vi "Gill_get_rdg.vi"(4 "Channel Name":string, 7 "Address":T1={"Main"=67, "Ch."=2, "Sub"=982, "Port Name"="Printer-Modem Port"}) -> (0 "Output":dbl format="%.2f", 3 "Status note":string)   [LabVIEW 2010]
uses:
  ADAM Client/Sub VIs/ADAM Controls/Address.ctl
  ADAM Client/Sub VIs/ADAM Controls/Remember_value_mode.ctl
panel:
  out "Concatenated String":string
  out "4521 Address":string
  out "Gill type":i32
  out "ADDRESS LETTER":string
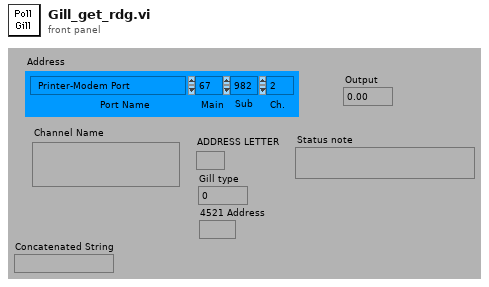
[diagram p1: front panel]
types:
  T1 = typedef "Address.ctl" = cluster{"Main":i32, "Ch.":i32, "Sub":i32, "Port Name":string}
  T2 = typedef "Remember_value_mode.ctl" = enum16{"Read only", "Read and Write"}
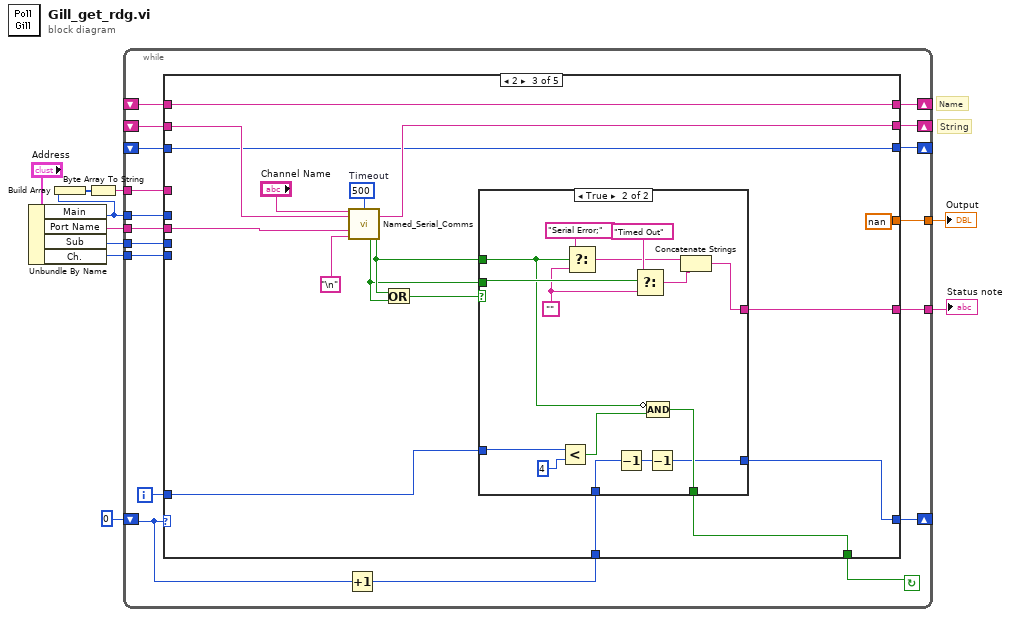
[diagram p0: block diagram]
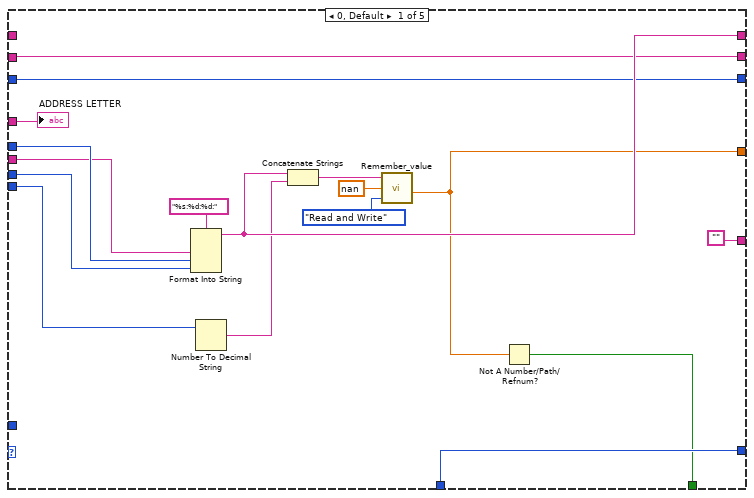
[diagram p2: hidden frame]
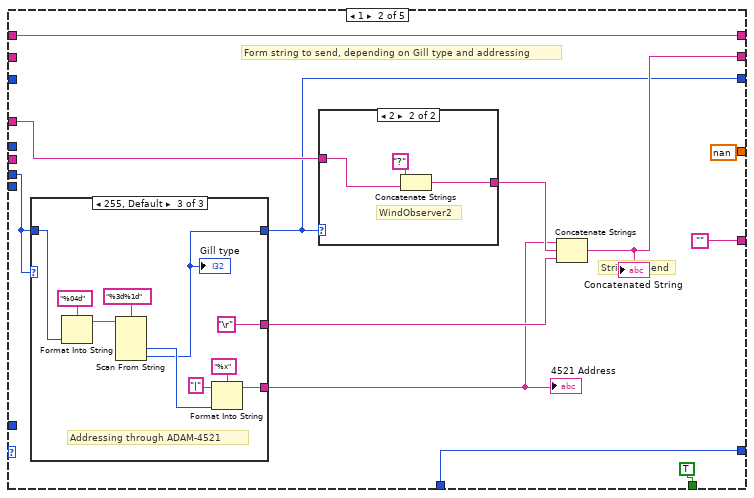
[diagram p3: hidden frame]
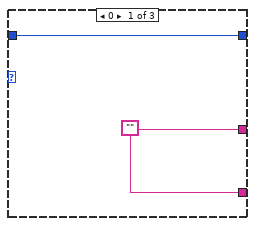
[diagram p4: hidden frame]
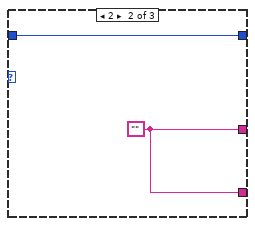
[diagram p5: hidden frame]
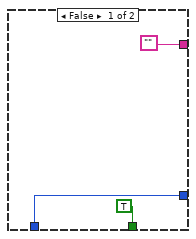
[diagram p7: hidden frame]
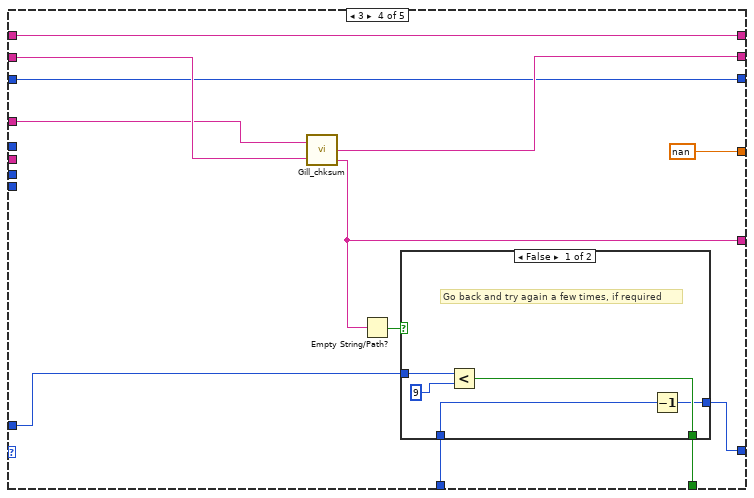
[diagram p8: hidden frame]
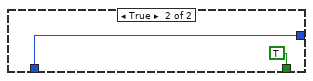
[diagram p9: hidden frame]
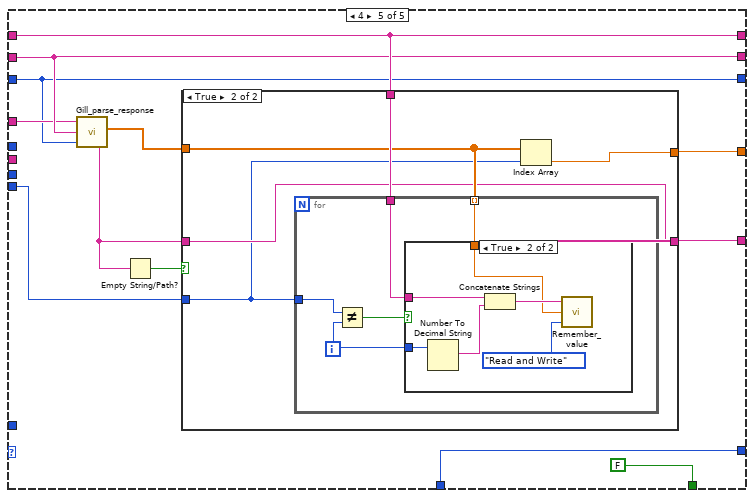
[diagram p10: hidden frame]
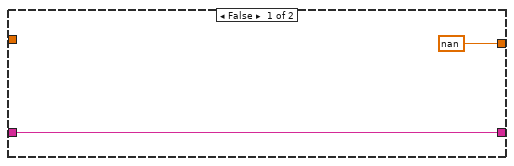
[diagram p11: hidden frame]
diagram:
  # "String"
  # "Name"
  n1 = Unbundle By Name("Address") -> ("Main"=w2:i32, "Port Name"=w9:string, "Sub"=w8:i32, "Ch."=w4:i32)
  n2 = Build Array(w2) -> (w3:i32[])
  n3 = Byte Array To String(unsigned byte array=w3) -> (string=w1:string)
  n4 = while {
    shift-left: _ -> [w11]
    shift-right: [w12] -> _
    tunnel: w1 -> [w13]
    shift-left: _ -> [w15]
    shift-right: [w16] -> _
    tunnel: [w19] -> w5
    tunnel: [w20] -> w6
    shift-left: _ -> [w14]
    shift-right: [w21] -> _
    shift-left: 0 -> [w24]
    shift-right: [w22] -> _
    tunnel: w4 -> [w25]
    tunnel: w2 -> [w26]
    tunnel: w8 -> [w27]
    tunnel: w9 -> [w28]
    i -> [w17]
    stop <- w18 continue-if-true
    n5 = Increment(x=w24) -> (x+1=w23:i32)
    n6 = case shown="2" w24 {
      tunnel: w28 -> [w31 _ w90 _ _]
      tunnel: w27 -> [w44 w53 _ _ _]
      tunnel: w26 -> [w45 _ _ _ _]
      tunnel: w25 -> [w42 _ _ _ w134]
      tunnel: w23 -> [w36 w46 w86 w113 w140]
      tunnel: [w36 w46 w85 w114 w140] -> w22
      tunnel: [w41 w55 w81 w119 w133] -> w21
      tunnel: [w33 nan nan nan w135] -> w20
      tunnel: ["" "" w89 w118 w141] -> w19
      tunnel: [w32 TRUE w83 w112 FALSE] -> w18
      tunnel: w17 -> [_ _ w84 w116 _]
      tunnel: [w35 w51 w82 w120 w132] -> w16
      tunnel: w15 -> [w35 _ w77 w121 w132]
      tunnel: w14 -> [_ w55 w81 w119 w133]
      tunnel: w13 -> [w30 w54 _ w117 w131]
      tunnel: [w29 w50 w76 w111 w130] -> w12
      tunnel: w11 -> [w29 _ w76 w111 w130]
      frame 0, Default {
        n7 = Format Into String(format string="%s:%d:%d:" ("Format String"), w31, w45, w44) -> (resulting string=w41:string)  [unwired: 2 in, 1 out]
        n8 = Number To Decimal String(number=w42) -> (decimal integer string=w40:string)  [unwired: 1 out]
        n9 = Concatenate Strings(w41, w40) -> (w39:string)
        n10 = call "Remember_value.vi"("Mode"=Remember_value_mode."Read and Write", "Input Value"=nan, "Ch name"=w39) -> ("Output Value"=w33:dbl)
        n11 = Not A Number/Path/Refnum?(number/path/refnum=w33) -> (NaN/Path/Refnum?=w32:bool)
        "ADDRESS LETTER" <- w30
      }
      frame 1 {
        # "Form string to send, depending on Gill type and addressing"
        # "String to send"
        n12 = case shown="255, Default" w53 {
          tunnel: [w59 w61 w62] -> w50
          tunnel: w53 -> [w59 w61 w71]
          tunnel: [w58 w60 w66] -> w48
          tunnel: [w58 w60 "\r"] -> w49
          frame 0 {
            w58 = ""
          }
          frame 2 {
            w60 = ""
          }
          frame 255, Default {
            # "Addressing through ADAM-4521"
            n13 = Format Into String(format string="%04d" ("Format String"), w71) -> (resulting string=w65:string)  [unwired: 2 in, 1 out]
            n14 = Scan From String(format string="%3d%1d" ("Format String"), input string=w65) -> (output 1=w63:i32, output 2=w62:i32)  [unwired: 2 in, 5 out]
            "Gill type" <- w62
            n15 = Format Into String(format string="%x" ("Format String"), initial string="|" ("Substring"), w63) -> (resulting string=w66:string)  [unwired: 1 in, 1 out]
          }
        }
        "4521 Address" <- w48
        n16 = case shown="2" w50 {
          tunnel: [w72 w74] -> w52
          tunnel: w54 -> [w72 w75]
          frame 0, Default {
            # "Original Gill"
          }
          frame 2 {
            # "WindObserver2"
            n17 = Concatenate Strings("?" ("Substring"), w75) -> (w74:string)
          }
        }
        n18 = Concatenate Strings(w48, w52, w49) -> (w51:string)
        "Concatenated String" <- w51
      }
      frame 2 {
        w92 = u32 500  # Timeout
        n19 = call "Named_Serial_Comms.vi"("Channel Name"="Channel Name", "Write String"=w77, "Timeout/ms"=w92, "Port Name"=w90, "Term Grep"="\n") -> ("Read"=w82:string, "Timed out"=w79:bool, "Serial Error"=w80:bool)  [unwired: 4 in, 4 out]
        n20 = Or(x=w80, y=w79) -> (x .or. y?=w87:bool)
        n21 = case shown="True" w87 {
          tunnel: ["" w109] -> w89
          tunnel: w80 -> [_ w98]
          tunnel: w79 -> [_ w110]
          tunnel: w86 -> [w94 w103]
          tunnel: [w94 w96] -> w85
          tunnel: w84 -> [_ w101]
          tunnel: [TRUE w97] -> w83
          frame False {
          }
          frame True {
            w104 = ""
            n22 = Less?(x=w101, y=4) -> (x < y?=w99:bool)
            n23 = Select(t="Serial Error;", s=w98, f=w104) -> (s? t:f=w106:string)
            n24 = Decrement(x=w103) -> (x-1=w102:i32)
            n25 = Select(t="Timed Out", s=w110, f=w104) -> (s? t:f=w105:string)
            n26 = Compound Arithmetic op=AND(invert w98, w99) -> (w97:bool)
            n27 = Decrement(x=w102) -> (x-1=w96:i32)
            n28 = Concatenate Strings(w106, w105) -> (w109:string)
          }
        }
      }
      frame 3 {
        n29 = call "Gill_chksum.vi"("Address"=w117, "Gill string"=w121) -> ("Stripped string"=w120:string, "Error Notes"=w118:string)  [unwired: 1 out]
        n30 = Empty String/Path?(string/path=w118) -> (empty?=w115:bool)
        n31 = case shown="False" w115 {
          tunnel: w116 -> [w126 _]
          tunnel: [w125 TRUE] -> w112
          tunnel: [w123 w128] -> w114
          tunnel: w113 -> [w124 w128]
          frame False {
            # "Go back and try again a few times, if required"
            n32 = Less?(x=w126, y=9) -> (x < y?=w125:bool)
            n33 = Decrement(x=w124) -> (x-1=w123:i32)
          }
          frame True {
          }
        }
      }
      frame 4 {
        n34 = call "Gill_parse_response.vi"("Address letter"=w131, "Stripped Gill response"=w132, "GILL TYPE NO."=w130) -> ("Numerics"=w139:dbl[], "Error notes"=w138:string)  [unwired: 2 out]
        n35 = Empty String/Path?(string/path=w138) -> (empty?=w137:bool)
        n36 = case shown="True" w137 {
          tunnel: [w142 w145] -> w141
          tunnel: w139 -> [_ w146]
          tunnel: [nan w148] -> w135
          tunnel: w138 -> [w142 w145]
          tunnel: w134 -> [_ w144]
          tunnel: w133 -> [_ w147]
          frame False {
          }
          frame True {
            n37 = for {
              tunnel: w147 -> [w153]
              tunnel: w146 -> [w152] mode=indexing
              tunnel: w144 -> [w150]
              i -> [w151]
              n38 = Not Equal?(x=w150, y=w151) -> (x != y?=w149:bool)
              n39 = case shown="True" w149 {
                tunnel: w151 -> [_ w159]
                tunnel: w153 -> [_ w157]
                tunnel: w152 -> [_ w154]
                frame False {
                }
                frame True {
                  n40 = Number To Decimal String(number=w159) -> (decimal integer string=w158:string)  [unwired: 1 out]
                  n41 = Concatenate Strings(w157, w158) -> (w155:string)
                  n42 = call "Remember_value.vi"("Mode"=Remember_value_mode."Read and Write", "Input Value"=w154, "Ch name"=w155) -> ()  [unwired: 1 out]
                }
              }
            }
            n43 = Index Array(array=w146, index=w144) -> (element=w148:dbl)
          }
        }
      }
    }
  }
  "Output" <- w6
  "Status note" <- w5
